vi "DoProcess.vi"(8 "error in (no error)":errorcluster, 9 "MsgQ":refnum<queue>, 10 "AbstractionActor.lvclass":refnum<class "AbstractionActor.lvclass">, 11 "ActionB in":refnum<class "ActionB.lvclass">) -> (0 "error out":errorcluster, 2 "AbstractionActor.lvclass 2":refnum<class "AbstractionActor.lvclass">, 3 "ActionB out":refnum<class "ActionB.lvclass">)   [LabVIEW 2014, in "ActionB.lvclass"]
uses:
  ActionB.lvclass
  RealWorkActor/RealWorkActor.lvclass
  AbstractionActor/AbstractionActor.lvclass
  AbstractionMessage/AbstractionMessage.lvclass
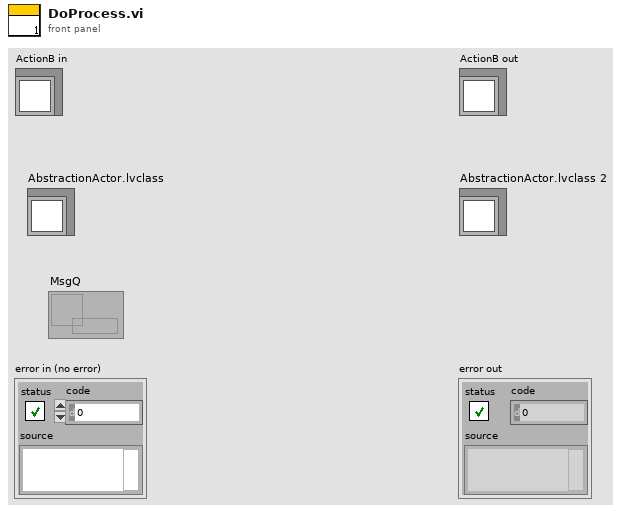
[diagram p1: front panel]
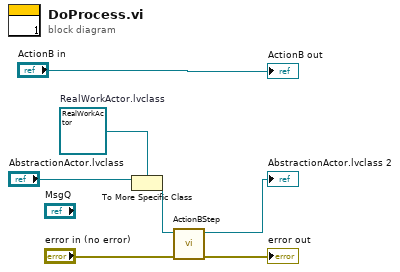
[diagram p0: block diagram]
diagram:
  w1 = refnum<class "RealWorkActor.lvclass"> refnum  # RealWorkActor.lvclass
  n1 = To More Specific Class(target class=w1, reference="AbstractionActor.lvclass") -> (specific class reference=w2:refnum<class "RealWorkActor.lvclass">)  [unwired: 1 in, 1 out]
  n2 = call "ActionBStep.vi"("error in (no error)"="error in (no error)", "RealWorkActor in"=w2) -> ("error out"=→"error out":errorcluster, "RealWorkActor out"=→"AbstractionActor.lvclass 2":refnum<class "RealWorkActor.lvclass">)  [unwired: 8 in]
  "ActionB out" <- "ActionB in"
